vi "Find Curvature Point.vi"(6 "Frame Number":i32, 7 "Min Curvature":dbl, 8 "error in (no error)":errorcluster, 9 "Search Direction":T4(ring), 10 "ROI Descriptor":T3 {"Contours"."Type" items=["No Selection", "Point", "Line", "Rectangle", "Oval", "Polygon", "Freehand Region", "Annulus", "Unused2", "Unused3", "Broken Line", "Freehand Line", "Rotated Rectangle"]}, 11 "Image":T5) -> (0 "error out":errorcluster, 2 "Tip":T1={"Point"={"X"=0.0, "Y"=0.0}, "Angle"=0.0, "Frame Number"=0, "ROI Descriptor"={"Global Rectangle"=[], "Contours"=[]}, "Curvature"=0.0, "Label"="Non-tip"} {"ROI Descriptor"."Contours"."Type" items=["No Selection", "Point", "Line", "Rectangle", "Oval", "Polygon", "Freehand Region", "Annulus", "Unused2", "Unused3", "Broken Line", "Freehand Line", "Rotated Rectangle"]; "Point"."Y" format="%.2f"; "Point"."X" format="%.2f"}, 3 "Image out":T5)   [LabVIEW 2013]
uses:
  <vilib>/vision/Image Controls.llb/IMAQ Image.ctl
  Controls/Tip.ctl
  <vilib>/vision/Contour.llb/IMAQ Connect Range Setting.ctl
  <vilib>/vision/Contour.llb/IMAQ Contour Curve Extraction.ctl
  <vilib>/vision/NI_Vision_Development_Module.lvlib
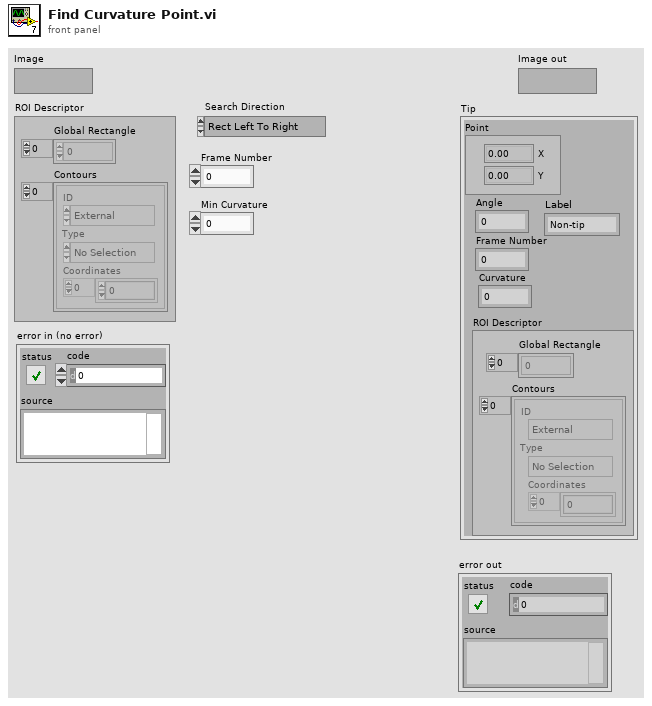
[diagram p1: front panel]
types:
  T1 = typedef "Tip.ctl" = cluster{"Point":T2, "Angle":dbl, "Frame Number":i32, "ROI Descriptor":T3, "Curvature":dbl, "Label":string}
  T2 = typedef "IMAQ Point" = cluster{"X":sgl, "Y":sgl}
  T3 = typedef "ROI Descriptor" = cluster{"Global Rectangle":i32[], "Contours":cluster{"ID":enum32{"External", "Internal"}, "Type":u32, "Coordinates":i32[]}[]}
  T4 = enum16{"Rect Left To Right", "Rect Right To Left", "Rect Top To Bottom", "Rect Bottom To Top", "Annulus Inner To Outer", "Annulus Outer To Inner", "Annulus Start Angle To End Angle", "Annulus End Angle To Start Angle"}
  T5 = typedef "IMAQ Image.ctl" = refnum<image>
  T6 = typedef "IMAQ Contour Curve Extraction.ctl" = cluster{"Extraction Mode":u32, "Edge Threshold":i32, "Edge Filter Size":u32, "Min Length":i32, "Search Step Size":i32, "Max Endpoint Gap":i32, "Subpixel":bool}
  T7 = typedef "IMAQ Connect Range Setting.ctl" = cluster{"Match Constraints":u32, "Min":dbl, "Max":dbl}
  T8 = enum16{"Closest To Search Start", "Maximum Length", "Strongest Mean Gradient Change"}
  T9 = typedef "IMAQ Rectangle" = cluster{"Left":i32, "Top":i32, "Right":i32, "Bottom":i32, "Rotation":dbl}
  T10 = cluster{"Overlay?":bool, "Color":u32, "Width":u32, "Maintain Width?":bool}
  T11 = cluster{"Point1 (Pixels)":cluster{"X":sgl, "Y":sgl}, "Point2 (Pixels)":cluster{"X":sgl, "Y":sgl}}
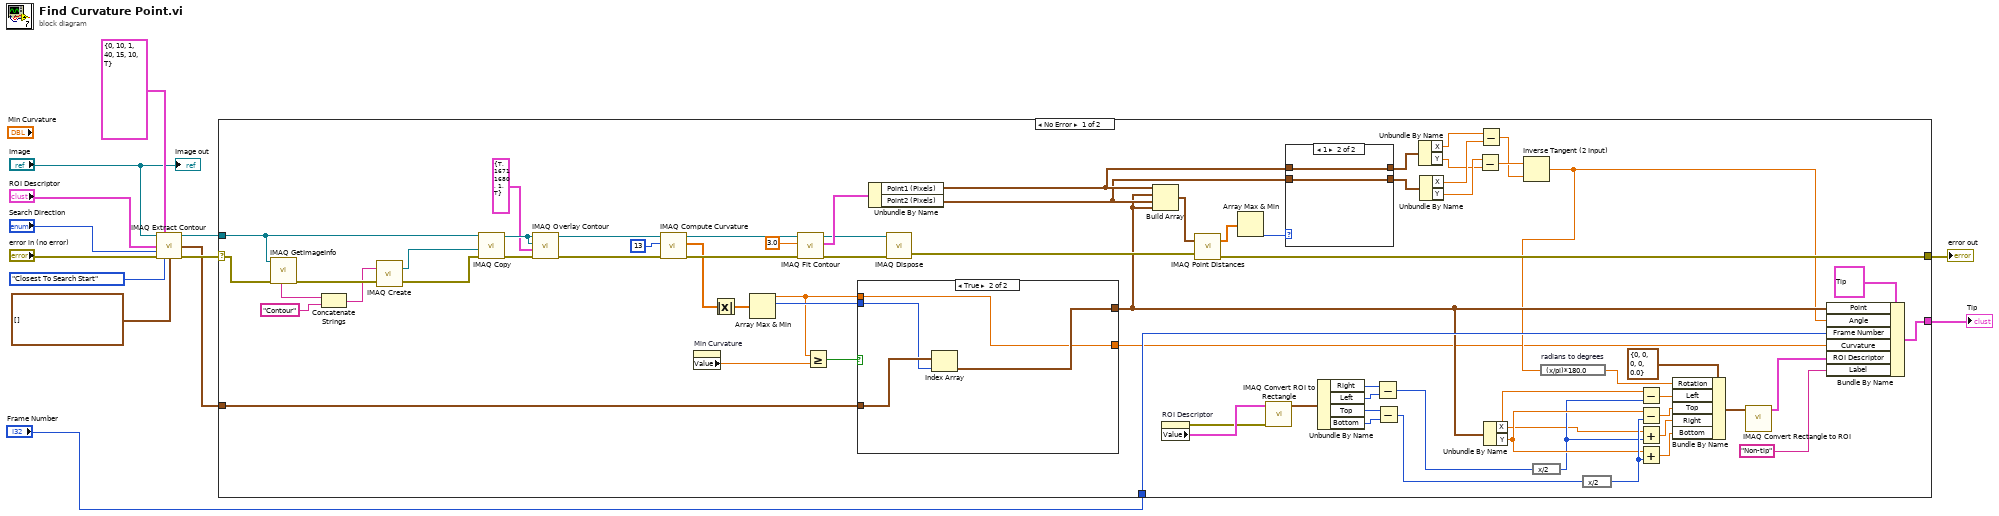
[diagram p0: block diagram]
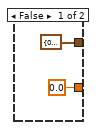
[diagram p3: hidden frame]
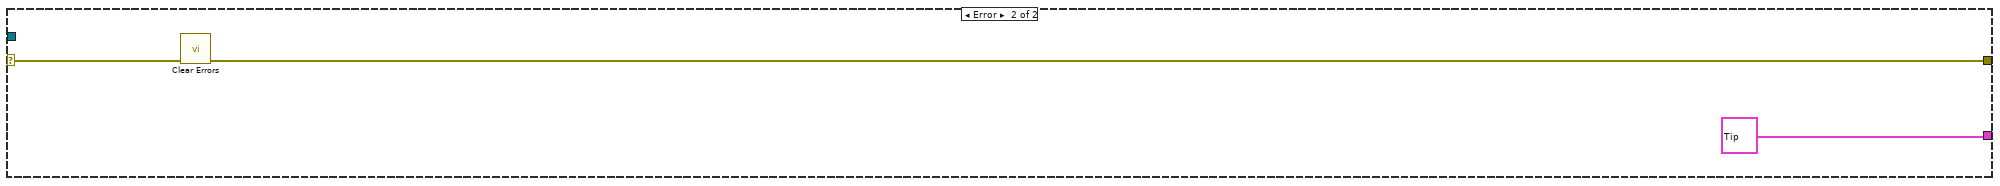
[diagram p4: hidden frame]
diagram:
  n1 = call "IMAQ Extract Contour"("Source Image"="Image", "Curve Extraction"=T6 {"Extraction Mode"=0, "Edge Threshold"=10, "Edge Filter Size"=1, "Min Length"=40, "Search Step Size"=15, "Max Endpoint Gap"=10, "Subpixel"=TRUE}, "ROI Descriptor"="ROI Descriptor", "Search Direction"="Search Direction", "error in (no error)"="error in (no error)", "Contour Selection"=T8."Closest To Search Start", "Curve Connection"=T7[] []) -> ("Source Image Out"=w7:T5, "Contour Points"=w4:cluster{"X":dbl, "Y":dbl}[], "error out"=w5:errorcluster)  [unwired: 1 in, 5 out]
  n2 = case shown="No Error" w5 {
    selector: w5 -> [w54 w96]
    tunnel: w7 -> [w53 _]
    tunnel: [w59 w95] -> w6
    tunnel: w4 -> [w72 _]
    tunnel: "Frame Number" -> [w74 _]
    tunnel: [w73 T1 {"Point"={"X"=0.0, "Y"=0.0}, "Angle"=0.0, "Frame Number"=0, "ROI Descriptor"={"Global Rectangle"=[], "Contours"=[]}, "Curvature"=0.0, "Label"=""} ("Tip")] -> w1
    frame No Error {
      n3 = call "IMAQ GetImageInfo"("error in (no error)"=w54, "Image"=w53) -> ("error out"=w52:errorcluster, "Image Name"=w56:string)  [unwired: 2 in, 6 out]
      n4 = Concatenate Strings(w56, "Contour" ("string")) -> (w51:string)
      n5 = call "IMAQ Create"("Image Name"=w51, "error in (no error)"=w52) -> ("New Image"=w49:T5, "error out"=w50:errorcluster)  [unwired: 3 in]
      n6 = call "IMAQ Copy"("error in (no error)"=w50, "Image Dst"=w49, "Image Src"=w53) -> ("error out"=w83:errorcluster, "Image Dst Out"=w82:T5)  [unwired: 3 in]
      n7 = call "IMAQ Overlay Contour"("error in (no error)"=w83, "Contour Points Settings"=T10 {"Overlay?"=TRUE, "Color"=16711680, "Width"=1, "Maintain Width?"=TRUE}, "Contour Image"=w82, "Image"=w82) -> ("error out"=w80:errorcluster, "Image Out"=w79:T5)  [unwired: 2 in, 4 out]
      n8 = call "IMAQ Compute Curvature"("error in (no error)"=w80, "Kernel Width"=u32 13, "Contour Image"=w79) -> ("error out"=w77:errorcluster, "Curvature Profile (pixel)"=w45:dbl[], "Contour Image Out (dup)"=w76:T5)  [unwired: 1 in, 5 out]
      n9 = property on="Min Curvature" class="DigNum (strict)"() -> ("Value"=w42:dbl)  [unwired: 2 in, 2 out]
      n10 = Absolute Value(x=w45) -> (abs(x)=w44:dbl[])
      n11 = Array Max & Min(array=w44) -> (max value=w41:dbl, max index (indices)=w43:i32)  [unwired: 2 out]
      n12 = call-poly "IMAQ Fit Contour"("error in (no error)"=w77, "Pixel Radius"=3.0, "Contour Image"=w76) -> ("error out"=w48:errorcluster, "Line Segment"=w71:T11, "Contour Image Out"=w47:T5)  [unwired: 1 in, 5 out]
      n13 = Greater Or Equal?(x=w41, y=w42) -> (x >= y?=w40:bool)
      n14 = case shown="True" w40 {
        tunnel: w72 -> [_ w93]
        tunnel: [cluster{"X":dbl, "Y":dbl} {"X"=0.0, "Y"=0.0} ("Point") w92] -> w27
        tunnel: w41 -> [_ w90]
        tunnel: w43 -> [_ w91]
        tunnel: [0.0 w90] -> w15
        frame False {
        }
        frame True {
          n15 = Index Array(array=w93, index=w91) -> (element=w92:cluster{"X":dbl, "Y":dbl})
        }
      }
      n16 = Unbundle By Name(w71) -> ("Point1 (Pixels)"=w67:cluster{"X":sgl, "Y":sgl}, "Point2 (Pixels)"=w66:cluster{"X":sgl, "Y":sgl})
      n17 = call "IMAQ Dispose"("Image"=w47, "error in (no error)"=w48) -> ("error out"=w46:errorcluster)  [unwired: 4 in]
      n18 = Build Array(w67, w27, w66, w27) -> (w70:cluster{"X":dbl, "Y":dbl}[])
      n19 = property on="ROI Descriptor" class="Clust (strict)"() -> (error out=w24:errorcluster, "Value"=w25:T3)  [unwired: 2 in, 1 out]
      n20 = call "IMAQ Point Distances"("Points"=w70, "error in (no error)"=w46) -> ("Distances"=w69:sgl[], "error out"=w59:errorcluster)  [unwired: 3 in]
      n21 = Array Max & Min(array=w69) -> (min index (indices)=w68:i32)  [unwired: 3 out]
      n22 = call "IMAQ Convert ROI to Rectangle"("error in (no error)"=w24, "ROI Descriptor"=w25) -> ("Rectangle"=w23:T9)  [unwired: 7 in, 1 out]
      n23 = case shown="1" w68 {
        tunnel: w67 -> [w84 w87]
        tunnel: w66 -> [w85 w86]
        tunnel: [w85 w87] -> w65
        tunnel: [w84 w86] -> w64
        frame 0, Default {
        }
        frame 1 {
        }
      }
      n24 = Unbundle By Name(w23) -> ("Right"=w22:i32, "Left"=w21:i32, "Top"=w20:i32, "Bottom"=w19:i32)
      n25 = Subtract(x=w22, y=w21) -> (x-y=w18:i32)
      n26 = Subtract(x=w20, y=w19) -> (x-y=w17:i32)
      n27 = Unbundle By Name(w65) -> ("X"=w63:sgl, "Y"=w57:sgl)
      n28 = Unbundle By Name(w64) -> ("X"=w62:sgl, "Y"=w58:sgl)
      n29 = Subtract(x=w58, y=w57) -> (x-y=w61:sgl)
      n30 = Subtract(x=w63, y=w62) -> (x-y=w60:sgl)
      n31 = Unbundle By Name(w27) -> ("X"=w28:dbl, "Y"=w30:dbl)
      n32 = Inverse Tangent (2 Input)(1:w60, 2:w61) -> (0:w26:sgl)
      n33 = expression code="x/2"(w18) -> (w29:i32)
      n34 = expression code="(x/pi)*180.0" "radians to degrees"(w26) -> (w37:sgl)
      n35 = expression code="x/2"(w17) -> (w31:i32)
      n36 = Subtract(x=w28, y=w29) -> (x-y=w34:dbl)
      n37 = Subtract(x=w30, y=w31) -> (x-y=w33:dbl)
      n38 = Add(x=w28, y=w29) -> (x+y=w36:dbl)
      n39 = Add(x=w30, y=w31) -> (x+y=w35:dbl)
      n40 = Bundle By Name(cluster=T9 {"Left"=0, "Top"=0, "Right"=0, "Bottom"=0, "Rotation"=0.0} ("Rectangle"), "Rotation"=w37, "Left"=w34, "Top"=w33, "Right"=w36, "Bottom"=w35) -> (w38:T9)
      n41 = call "IMAQ Convert Rectangle to ROI"("Rectangle"=w38) -> ("ROI Descriptor"=w16:T3)  [unwired: 8 in, 1 out]
      n42 = Bundle By Name(cluster=T1 {"Point"={"X"=0.0, "Y"=0.0}, "Angle"=0.0, "Frame Number"=0, "ROI Descriptor"={"Global Rectangle"=[], "Contours"=[]}, "Curvature"=0.0, "Label"=""} ("Tip"), "Point"=w27, "Angle"=w26, "Frame Number"=w74, "Curvature"=w15, "ROI Descriptor"=w16, "Label"="Non-tip") -> (w73:T1)
    }
    frame Error {
      n43 = call <vilib>:"Clear Errors.vi"("error in (no error)"=w96) -> ("error out"=w95:errorcluster)  [unwired: 6 in]
    }
  }
  "error out" <- w6
  "Tip" <- w1
  "Image out" <- "Image"
